vi "Identifier.vi"(11 "User in":refnum<class "User.lvclass">) -> (2 "Identifier":refnum<class "String.lvclass">)   [LabVIEW 2020, in "HTTP-Conditum.lvlib" / "User.lvclass"]
uses:
  User.lvclass
  <vilib>/IlluminatedG/IG Conditum/Conditum/Columns/String/String.lvclass
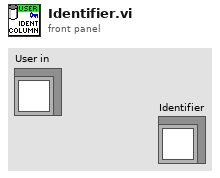
[diagram p1: front panel]
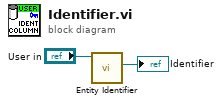
[diagram p0: block diagram]
diagram:
  n1 = call-dynamic "Entity Identifier.vi"("User in"="User in") -> ("Identifier Column"=→"Identifier":refnum<class "String.lvclass">)  [unwired: 10 in]
